vi "Vol-Play.vi"(6 "State":T2, 7 "Cycle number (in)":i32, 8 "error in (no error)":errorcluster, 10 "Stop button pressed":bool, 11 "Number of Frames":u32) -> (0 "error out":errorcluster, 1 "Cycle number (out)":i32, 2 "Speed data waveform graph":dbl[](graph), 3 "I mage ref out":T1, 4 "Playback stopped":bool, 5 "Image Array":T1[](array[typedef]))   [LabVIEW 2020]
uses:
  <vilib>/vision/Image Controls.llb/IMAQ Image.ctl
  Timelapse Viewer/Typedefs/Speed Viewer States enum.ctl
  Timelapse Viewer/Typedefs/Select Play-Stop button to show.ctl
  Timelapse Viewer/Globals/gl_Time series viewer globals.vi
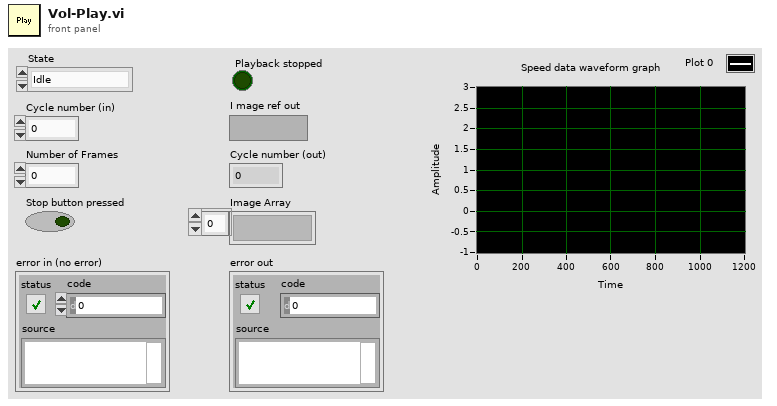
[diagram p1: front panel]
types:
  T1 = typedef "IMAQ Image.ctl" = refnum<image>
  T2 = typedef "Speed Viewer States enum.ctl" = enum16{"Idle", "Initialise", "Playback", "Scroll bar event", "Speed cursor event", "Back to start", "Exit"}
  T3 = typedef "Time series viewer refs.ctl" = cluster{"This VI":refnum<vi>, "Image control":refnum<vi>, "AVI Mode ind":refnum<vi>, "Play":refnum<vi>, "Stop":refnum<vi>, "Back":refnum<vi>, "Scrollbar":refnum<vi>, "Video length info":refnum<vi>, "Expected speed values":refnum<vi>, "Intensity":refnum<vi>, "Path":refnum<vi>, "Selection sliders":refnum<vi>, "Speed Graph ref":refnum<vi>, "Frame rate set (fps)":refnum<vi>, "Number of rows to generate":refnum<vi>, "VL Image Array":refnum<vi>, "Image Scrollbar":refnum<vi>, "Channel to load":refnum<vi>, "Colour":refnum<vi>}
  T4 = typedef "Channel to load.ctl" = enum16{"Show red channel", "Show green channel", "Show both channels"}
  T5 = typedef "Select Play-Stop button to show.ctl" = enum16{"Show Play button", "Show Stop button"}
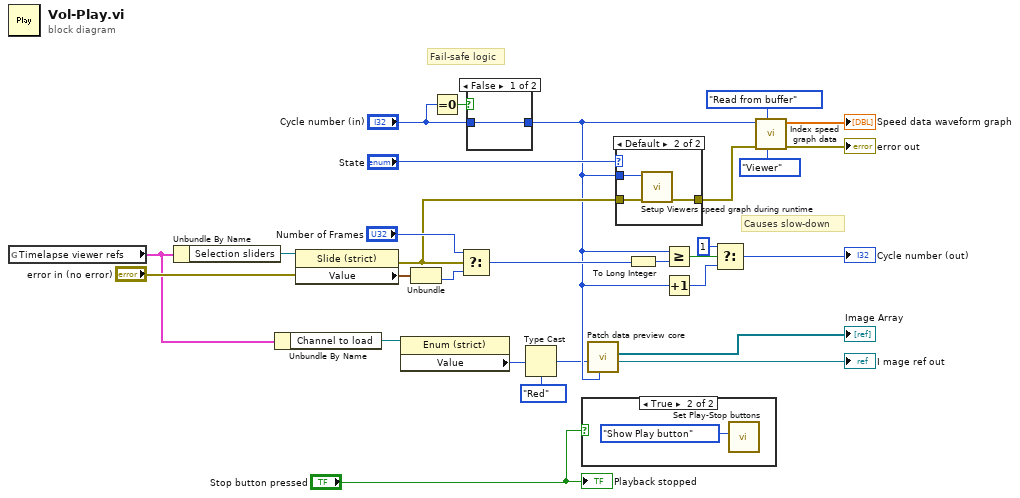
[diagram p0: block diagram]
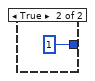
[diagram p4: hidden frame]
diagram:
  # "Causes slow-down"
  # "Fail-safe logic"
  n1 = global read "gl_Time series viewer globals.vi" "Timelapse viewer refs"() -> (w11:T3)
  n2 = Unbundle By Name(w11) -> ("Selection sliders"=w22:refnum<vi>)
  n3 = Unbundle By Name(w11) -> ("Channel to load"=w10:refnum<vi>)
  n4 = property class="Slide (strict)"(reference=w22, error in="error in (no error)") -> (error out=w14:errorcluster, "Value"=w21:cluster{i32, i32})  [unwired: 1 out]
  n5 = property class="Enum (strict)"(reference=w10) -> ("Value"=w5:T4)  [unwired: 1 in, 2 out]
  n6 = Unbundle(w21) -> (w20:i32)  [unwired: 1 out]
  n7 = Equal To 0?(x="Cycle number (in)") -> (x = 0?=w8:bool)
  n8 = Select(t="Number of Frames", s=w14, f=w20) -> (s? t:f=w19:u32)
  n9 = case shown="False" w8 {
    tunnel: [w30 1 ("Value")] -> w6
    tunnel: "Cycle number (in)" -> [w30 _]
    frame False {
    }
    frame True {
    }
  }
  n10 = Type Cast(type=enum16{"Red", "Green"}."Red" ("Channel to load"), x=w5) -> (*(type *) &x=w4:enum16{"Red", "Green"})
  n11 = case shown="True" "Stop button pressed" {
    frame False {
    }
    frame True {
      n12 = call "Set Play-Stop buttons.vi"("Function"=Select_Play-Stop_button_to_show."Show Play button") -> ()  [unwired: 10 in, 1 out]
    }
  }
  n13 = call "Patch data preview core.vi"("Global cycle number among all trials"=w6, "Channel to load"=w4) -> ("Image ref (montage)"=→"I mage ref out":T1, "Array"=→"Image Array":T1[])  [unwired: 7 in, 1 out]
  n14 = case shown="Default" "State" {
    tunnel: w14 -> [w33 w36]
    tunnel: [w33 w35] -> w13
    tunnel: w6 -> [_ w34]
    frame "Speed cursor event" {
    }
    frame Default {
      n15 = call "Setup Viewers speed graph during runtime.vi"("error in (no error)"=w36, "Frame number or cycle number"=w34) -> ("error out"=w35:errorcluster)  [unwired: 9 in]
    }
  }
  n16 = To Long Integer(number=w19) -> (32bit integer=w24:i32)
  n17 = Greater Or Equal?(x=w6, y=w24) -> (x >= y?=w28:bool)
  n18 = Increment(x=w6) -> (x+1=w29:i32)
  n19 = Select(t=1, s=w28, f=w29) -> (s? t:f=→"Cycle number (out)":i32)
  n20 = call "Index speed graph data.vi"("Caller"=enum16{"Viewer", "Exporter"}."Viewer", "Buffer operation (read from internal buffer)"=enum16{"Update buffer", "Read from buffer"}."Read from buffer", "error in (no error)"=w13, "Gobal frame number in Timelapse data/master video (1 based)"=w6) -> ("error out"=→"error out":errorcluster, "Speed data waveform graph"=→"Speed data waveform graph":dbl[])  [unwired: 5 in, 1 out]
  "Playback stopped" <- "Stop button pressed"
